vi "Exercise 1.5 Read GPIO PWM.vi"(8 "error in (no error)":errorcluster) -> (0 "error out":errorcluster)   [LabVIEW 2014]
uses:
  <vilib>/Q-Wave Systems/QwaveSys RPi Training Package (Demo)/Addons/QwaveSys RPi Training Library.lvlib
  <vilib>/Q-Wave Systems/QwaveSys RPi Training Package (Demo)/Addons/WiringPi/WiringPi Pin Mode.ctl
  <vilib>/Q-Wave Systems/QwaveSys RPi Training Package (Demo)/Addons/WiringPi/WiringPi PullUpDown.ctl
  <vilib>/Q-Wave Systems/QwaveSys RPi Training Package (Demo)/Addons/WiringPi/WiringPi GPIO TypeDef.ctl
panel:
  in  "Button":T1=7 items=["Pin1_3.3V"=51, "Pin2_5V"=52, "Pin3_GPIO8_I2C1_SDA"=8, "Pin4_5V"=53, "Pin5_GPIO9_I2C1_SCL"=9, "Pin6_Gnd"=54, "Pin7_GPIO7_GPCLK0"=7, "Pin8_GPIO15_TXD_UART"=15, "Pin9_Gnd"=55, "Pin10_GPIO16_RXD_UART"=16, "Pin11_GPIO0"=0, "Pin12_GPIO1_PCMCLK_PWM0"=1, "Pin13_GPIO2"=2, "Pin14_Gnd"=56, "Pin15_GPIO3"=3, "Pin16_GPIO4"=4, "Pin17_3V"=57, "Pin18_GPIO5"=5, "Pin19_GPIO12_MOSI(SPI)"=12, "Pin20_Gnd"=58, "Pin21_GPIO13_MISO(SPI)"=13, "Pin22_GPIO6"=6, "Pin23_GPIO14_CLK(SPI)"=14, "Pin24_GPIO10_CE0_SPI"=10, "Pin25_Gnd"=59, "Pin26_GPIO11_CE1_SPI"=11, "Pin27_SDA0_I2C_EEPROM"=60, "Pin28_SCL0_I2C_EEPROM"=61, "Pin_29_GPIO21_GPCLK1"=21, "Pin30_Gnd"=62, "Pin31_GPIO22_GPCLK2"=22, "Pin32_GPIO26_PWM0"=26, "Pin33_GPIO23_PWM1"=23, "Pin34_Gnd"=63, "Pin35_GPIO24_PCMFS_PWM1"=24, "Pin36_GPIO27"=27, "Pin37_GPIO25"=25, "Pin38_GPIO28_PCM_DIN"=28, "Pin39_Gnd"=64, "Pin40_GPIO29_PCM_DOUT"=29]
  in  "LED":T1=1 items=["Pin1_3.3V"=51, "Pin2_5V"=52, "Pin3_GPIO8_I2C1_SDA"=8, "Pin4_5V"=53, "Pin5_GPIO9_I2C1_SCL"=9, "Pin6_Gnd"=54, "Pin7_GPIO7_GPCLK0"=7, "Pin8_GPIO15_TXD_UART"=15, "Pin9_Gnd"=55, "Pin10_GPIO16_RXD_UART"=16, "Pin11_GPIO0"=0, "Pin12_GPIO1_PCMCLK_PWM0"=1, "Pin13_GPIO2"=2, "Pin14_Gnd"=56, "Pin15_GPIO3"=3, "Pin16_GPIO4"=4, "Pin17_3V"=57, "Pin18_GPIO5"=5, "Pin19_GPIO12_MOSI(SPI)"=12, "Pin20_Gnd"=58, "Pin21_GPIO13_MISO(SPI)"=13, "Pin22_GPIO6"=6, "Pin23_GPIO14_CLK(SPI)"=14, "Pin24_GPIO10_CE0_SPI"=10, "Pin25_Gnd"=59, "Pin26_GPIO11_CE1_SPI"=11, "Pin27_SDA0_I2C_EEPROM"=60, "Pin28_SCL0_I2C_EEPROM"=61, "Pin_29_GPIO21_GPCLK1"=21, "Pin30_Gnd"=62, "Pin31_GPIO22_GPCLK2"=22, "Pin32_GPIO26_PWM0"=26, "Pin33_GPIO23_PWM1"=23, "Pin34_Gnd"=63, "Pin35_GPIO24_PCMFS_PWM1"=24, "Pin36_GPIO27"=27, "Pin37_GPIO25"=25, "Pin38_GPIO28_PCM_DIN"=28, "Pin39_Gnd"=64, "Pin40_GPIO29_PCM_DOUT"=29]
  out "PWM RAW Output":i32(knob)=862 scale=0.0..300.0
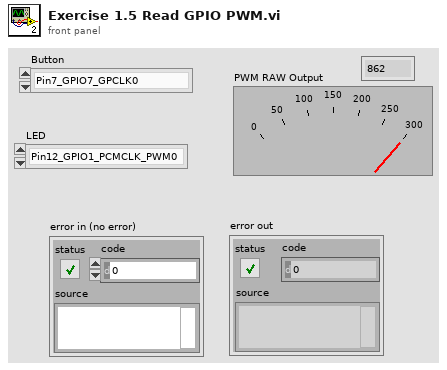
[diagram p1: front panel]
types:
  T1 = typedef "QwaveSys RPi Training Library.lvlib/WiringPi GPIO TypeDef.ctl" = u8
  T2 = typedef "QwaveSys RPi Training Library.lvlib/WiringPi Pin Mode.ctl" = enum8{"INPUT", "OUTPUT", "PWM_OUTPUT", "GPIO_CLOCK", "SOFT_PWM_OUTPUT", "SOFT_TONE_OUTPUT", "PWM_TONE_OUTPUT"}
  T3 = typedef "QwaveSys RPi Training Library.lvlib/WiringPi PullUpDown.ctl" = enum8{"PUD_OFF", "PUD_DOWN", "PUD_UP"}
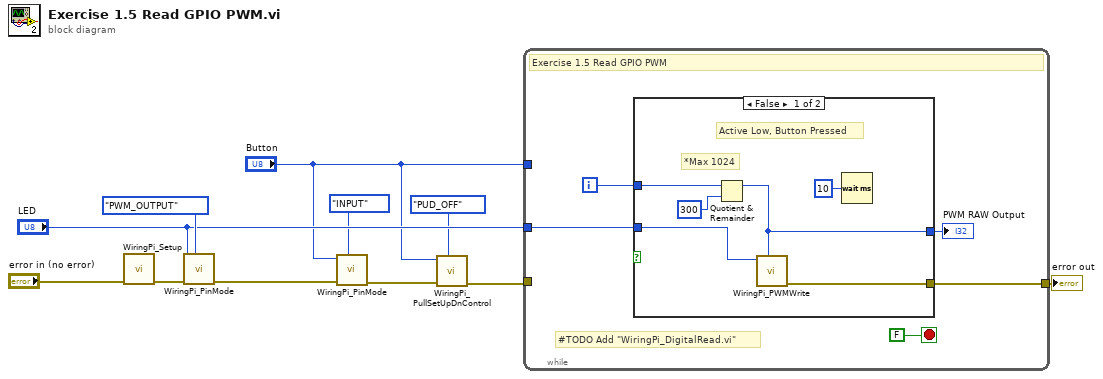
[diagram p0: block diagram]
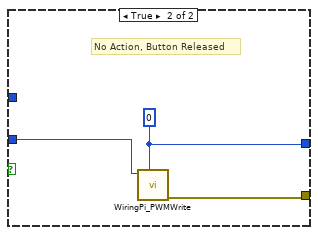
[diagram p2: hidden frame]
diagram:
  n1 = call <vilib>:"WiringPi_Setup.vi"("error in (no error)"="error in (no error)") -> ("error out"=w10:errorcluster)  [unwired: 10 in]
  n2 = call <vilib>:"WiringPi_PinMode.vi"("Pin Mode"=WiringPi_Pin_Mode."PWM_OUTPUT", "error in (no error)"=w10, "WiringPi GPIO"="LED") -> ("error out"=w7:errorcluster)  [unwired: 8 in]
  n3 = call <vilib>:"WiringPi_PinMode.vi"("Pin Mode"=WiringPi_Pin_Mode."INPUT", "error in (no error)"=w7, "WiringPi GPIO"="Button") -> ("error out"=w5:errorcluster)  [unwired: 8 in]
  n4 = call <vilib>:"WiringPi_PullSetUpDnControl.vi"("Pull Up Down Mode"=WiringPi_PullUpDown."PUD_OFF", "error in (no error)"=w5, "WiringPi GPIO"="Button") -> ("error out"=w3:errorcluster)  [unwired: 8 in]
  n5 = while {
    tunnel: w3 -> [_]
    tunnel: "LED" -> [w14]
    tunnel: "Button" -> [_]
    tunnel: [w13] -> w1
    i -> [w15]
    stop <- FALSE stop-if-true
    # "#TODO Add \"WiringPi_DigitalRead.vi\""
    # "Exercise 1.5 Read GPIO PWM"
    n6 = case shown="False" {
      selector: _ -> [_ _]
      tunnel: w15 -> [w20 _]
      tunnel: w14 -> [w19 w24]
      tunnel: [w18 w25] -> w13
      tunnel: [w17 w23] -> w12
      frame False {
        # "Active Low, Button Pressed"
        # "*Max 1024"
        n7 = Quotient & Remainder(x=w20, y=300) -> (x-y*floor(x/y)=w17:i32)  [unwired: 1 out]
        n8 = call <vilib>:"WiringPi_PWMWrite.vi"("Value"=w17, "WiringPi GPIO"=w19) -> ("error out"=w18:errorcluster)  [unwired: 9 in]
        n9 = Wait (ms)(milliseconds to wait=u32 10) -> ()  [unwired: 1 out]
      }
      frame True {
        w23 = 0 ("Value")
        # "No Action, Button Released"
        n10 = call <vilib>:"WiringPi_PWMWrite.vi"("Value"=w23, "WiringPi GPIO"=w24) -> ("error out"=w25:errorcluster)  [unwired: 9 in]
      }
    }
    "PWM RAW Output" <- w12
  }
  "error out" <- w1
